vi "Importing FFT Data class VI - retrieve data.vi"(8 "error in (no error)":errorcluster, 11 "Imported FFT Data in":refnum<class "Imported FFT Data.lvclass">) -> (0 "error out":errorcluster, 1 "Array 2":dbl[][](array[numeric]), 2 "Array":dbl[][](array[numeric]), 3 "Imported FFT Data out":refnum<class "Imported FFT Data.lvclass">, 4 "FFTs Table":string[][](array[string]), 5 "Row":i32)   [LabVIEW 2010, in "Imported FFT Data.lvclass"]
uses:
  Imported FFT Data.lvclass
  Imported FFT Data.lvclass/Imported FFT Data.ctl
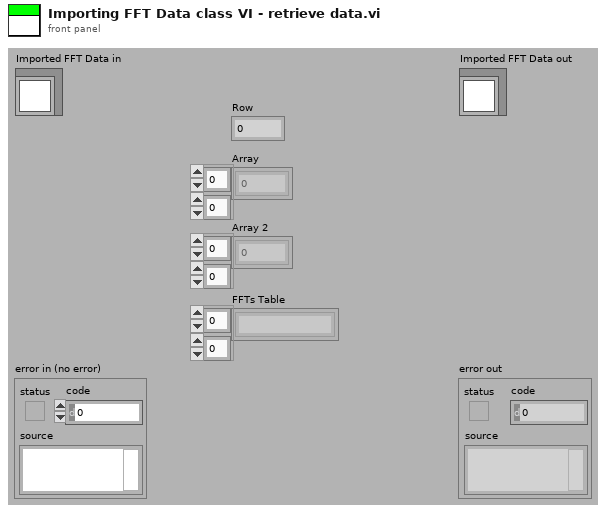
[diagram p1: front panel]
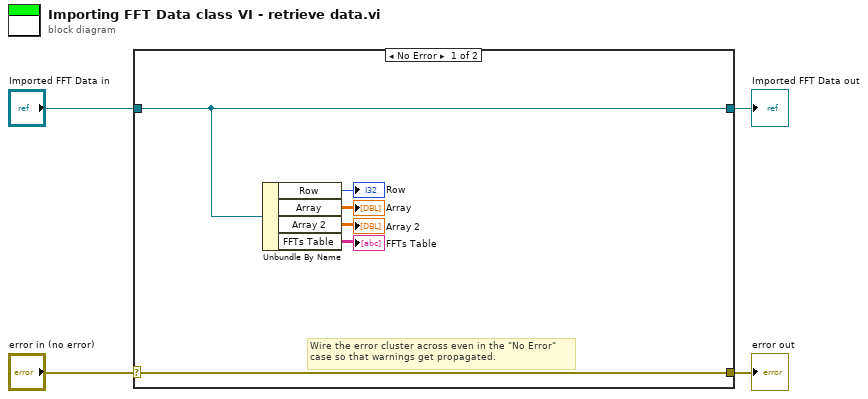
[diagram p0: block diagram]
diagram:
  n1 = case shown="No Error" "error in (no error)" {
    selector: "error in (no error)" -> [w10 w12]
    tunnel: [w10 w12] -> w3
    tunnel: [w9 w11] -> w1
    tunnel: "Imported FFT Data in" -> [w9 w11]
    frame No Error {
      # "Wire the error cluster across even in the \"No Error\"\ncase so that warnings get propagated."
      n2 = Unbundle By Name(w9) -> ("Row"=→"Row":i32, "Array"=→"Array":dbl[][], "Array 2"=→"Array 2":dbl[][], "FFTs Table"=→"FFTs Table":string[][])
    }
    frame Error {
    }
  }
  "error out" <- w3
  "Imported FFT Data out" <- w1
